vi "CreateWriteCluster.vi"(2 "Page Size in Bytes":u32=128, 3 "EEPROM Starting Address":u16, 4 "Number of Bytes to Write":u32=128) -> (0 "Array of Write Cluster Information":T1(array[cluster]))   [LabVIEW 2025]
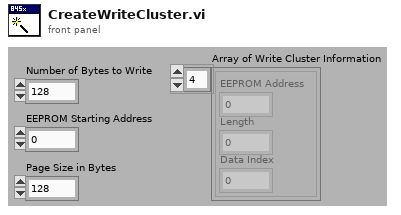
[diagram p1: front panel]
types:
  T1 = cluster{"EEPROM Address":u16, "Length":u32, "Data Index":u32}[]
  T2 = cluster{"EEPROM Address":u16, "Length":u32, "Data Index":u32}
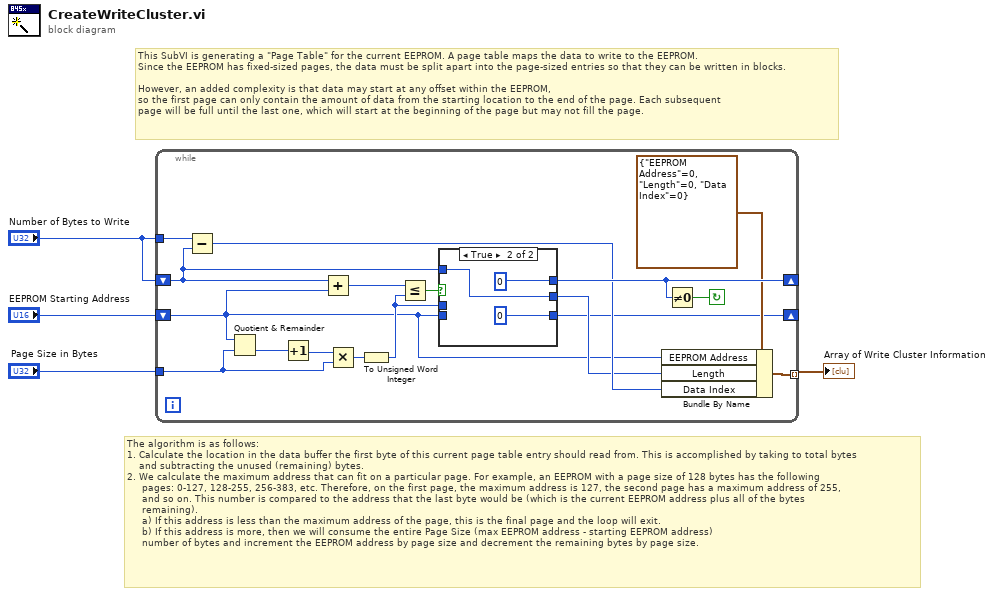
[diagram p0: block diagram]
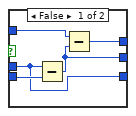
[diagram p2: hidden frame]
diagram:
  # "The algorithm is as follows:\n1. Calculate the location in the data buffer the first byte of this current page table entry should read from. This is accomplished by taking to total bytes \n    and subtracting the unused (remaining) bytes.\n2. We calculate the maximum address that can fit on a particular page. For example, an EEPROM with a page size of 128 bytes has the following   \n     pages: 0-127, 128-255, 256-383, etc. Therefore, on the first page, the maximum address is 127, the second page has a maximum address of 255, \n     and so on. This number is compared to the address that the last byte would be (which is the current EEPROM address plus all of the bytes \n     remaining). \n     a) If this address is less than the maximum address of the page, this is the final page and the loop will exit.  \n     b) If this address is more, then we will consume the entire Page Size (max EEPROM address - starting EEPROM address)\n     number of bytes and increment the EEPROM address by page size and decrement the remaining bytes by page size."
  # "This SubVI is generating a \"Page Table\" for the current EEPROM. A page table maps the data to write to the EEPROM. \nSince the EEPROM has fixed-sized pages, the data must be split apart into the page-sized entries so that they can be written in blocks.\n\nHowever, an added complexity is that data may start at any offset within the EEPROM, \nso the first page can only contain the amount of data from the starting location to the end of the page. Each subsequent  \npage will be full until the last one, which will start at the beginning of the page but may not fill the page."
  n1 = while {
    tunnel: "Number of Bytes to Write" -> [w15]
    shift-right: [w13] -> _
    shift-left: "Number of Bytes to Write" -> [w14]
    shift-right: [w7] -> _
    shift-left: "EEPROM Starting Address" -> [w8]
    tunnel: [w10] -> w2 mode=indexing
    tunnel: "Page Size in Bytes" -> [w5]
    stop <- w6 continue-if-true
    n2 = Subtract(x=w15, y=w14) -> (x-y=w12:u32)
    n3 = Quotient & Remainder(x=w8, y=w5) -> (floor(x/y)=w21:u32)  [unwired: 1 out]
    n4 = Increment(x=w21) -> (x+1=w20:u32)
    n5 = Add(x=w14, y=w8) -> (x+y=w18:u32)
    n6 = Multiply(x=w20, y=w5) -> (x*y=w19:u32)
    n7 = To Unsigned Word Integer(number=w19) -> (unsigned 16bit integer=w16:u16)
    n8 = Less Or Equal?(x=w18, y=w16) -> (x <= y?=w17:bool)
    n9 = case shown="True" w17 {
      tunnel: [w24 u32 0] -> w13
      tunnel: w16 -> [w22 _]
      tunnel: w8 -> [w26 _]
      tunnel: w14 -> [w25 w27]
      tunnel: [w22 u16 0] -> w7
      tunnel: [w23 w27] -> w9
      frame False {
        n10 = Subtract(x=w22, y=w26) -> (x-y=w23:u16)
        n11 = Subtract(x=w25, y=w23) -> (x-y=w24:u32)
      }
      frame True {
      }
    }
    n12 = Bundle By Name(cluster=T2 {"EEPROM Address"=0, "Length"=0, "Data Index"=0}, "EEPROM Address"=w8, "Length"=w9, "Data Index"=w12) -> (w10:T2)
    n13 = Not Equal To 0?(x=w13) -> (x != 0?=w6:bool)
  }
  "Array of Write Cluster Information" <- w2
